vi "svc_Build Unit Label for Frequency Range.vi"(7 "number of decimal places to add":i32 min=0 max=32, 9 "x-axis unit label":string="Hz", 10 "fmax":dbl=20000.0 format="%.2f", 11 "f0":dbl=20.0 format="%.2f") -> (3 "frequency range string":string)   [LabVIEW 2017]
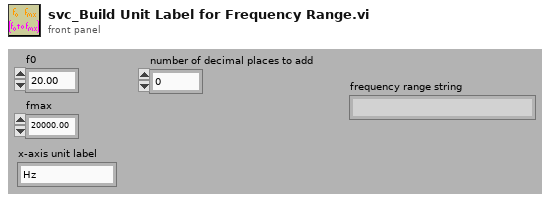
[diagram p1: front panel]
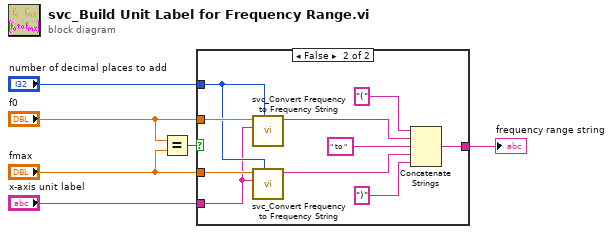
[diagram p0: block diagram]
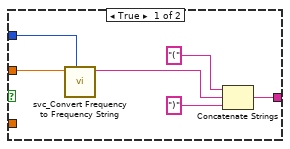
[diagram p2: hidden frame]
diagram:
  n1 = Equal?(x="f0", y="fmax") -> (x = y?=w2:bool)
  n2 = case shown="False" w2 {
    tunnel: [w12 w22] -> w6
    tunnel: "f0" -> [w10 w19]
    tunnel: "fmax" -> [_ w17]
    tunnel: "number of decimal places to add" -> [w8 w15]
    tunnel: "x-axis unit label" -> [_ w13]
    frame True {
      n3 = call <vilib>:"svc_Convert Frequency to Frequency String.vi"("number of decimal places to add"=w8, "frequency [Hz]"=w10) -> ("frequency string"=w9:string)  [unwired: 9 in]
      n4 = Concatenate Strings("(", w9, ")") -> (w12:string)
    }
    frame False {
      n5 = call <vilib>:"svc_Convert Frequency to Frequency String.vi"("number of decimal places to add"=w15, "x-axis unit label"=w13, "frequency [Hz]"=w19) -> ("frequency string"=w18:string)  [unwired: 8 in]
      n6 = call <vilib>:"svc_Convert Frequency to Frequency String.vi"("number of decimal places to add"=w15, "x-axis unit label"=w13, "frequency [Hz]"=w17) -> ("frequency string"=w16:string)  [unwired: 8 in]
      n7 = Concatenate Strings("(", w18, " to ", w16, ")") -> (w22:string)
    }
  }
  "frequency range string" <- w6
